vi "PSOCE_Protocol.vi"(0 "y_center":dbl, 1 "y_span":dbl, 2 "mode":i32=50, 3 "galvo phase":i32, 4 "x_center":dbl, 5 "x_span":dbl=5.0, 6 "n_lines":i32=50, 9 "flyback_lines":i32=4, 10 "n frames":i32=20, 11 "Custom trig.":T1={"n_frames to c. trig"=1, "custom trig length (frames)"=1, "n_frames between c. trig"=1, "n_custom trigger"=1}) -> (14 "x_data":dbl[](graph), 15 "y_data":dbl[](graph), 17 "trigger out":u32[](graph), 18 "custom trig out":u32[](graph), 19 "Overall Frames":i32)   [LabVIEW 2021]
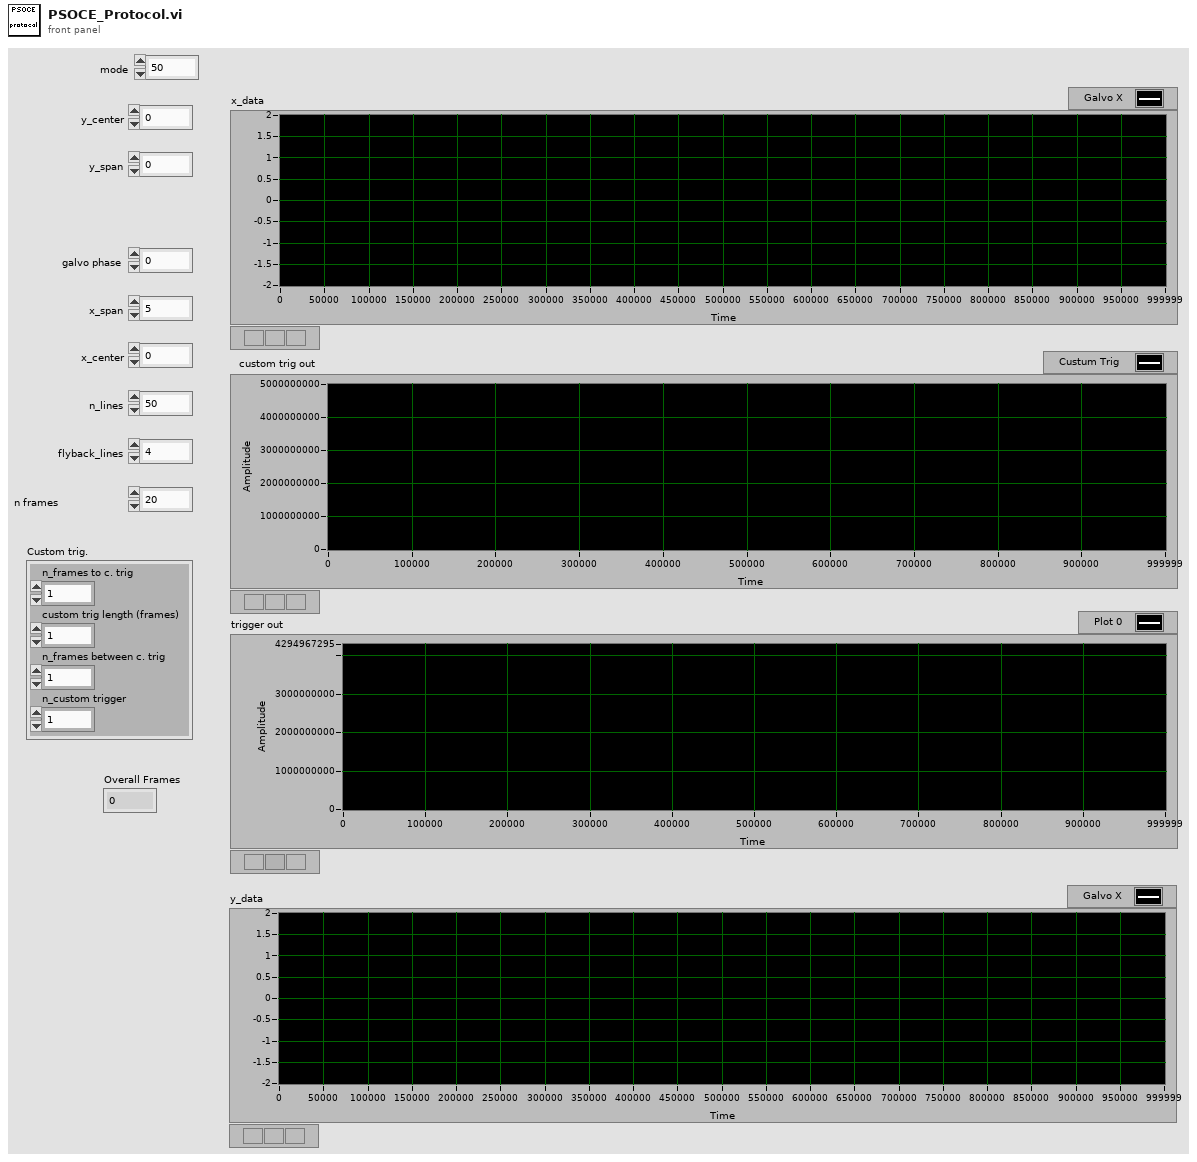
[diagram p1: front panel]
types:
  T1 = cluster{"n_frames to c. trig":i32, "custom trig length (frames)":i32, "n_frames between c. trig":i32, "n_custom trigger":i32}
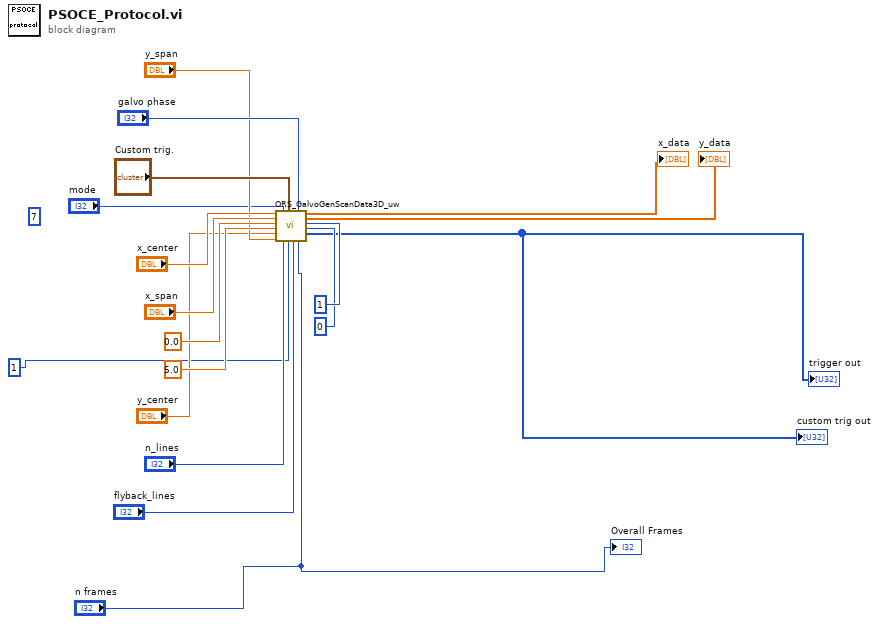
[diagram p0: block diagram]
diagram:
  (unwired) 7 ("mode")
  n1 = call "ORS_GalvoGenScanData3D_uw.vi"("x_center"="x_center", "x_span"="x_span", "offset"=0.0, "span-factor"=5.0, "y_center"="y_center", "y_span"="y_span", "mode"="mode", "n_lines"="n_lines", "Custom trig."="Custom trig.", "n_frames same y pos"=u32 1 ("n_3D scans"), "flyback_lines"="flyback_lines", "galvo phase"="galvo phase", "n_frames"="n frames", "n_3D scans"=u32 1, "flyback frames"=u16 0) -> ("x_data"=→"x_data":dbl[], "y_data"=→"y_data":dbl[], "trigger out"=→"custom trig out" →"trigger out":u32[])  [unwired: 2 out]
  "Overall Frames" <- "n frames"
